vi "Configurable PWM Pulse Time Tester.vi"() -> ()   [LabVIEW 2021]
uses:
  <vilib>/Utility/error.llb/DialogType.ctl
  <vilib>/DAQmx/write.llb/DAQmx Write (Counter Frequency 1Chan 1Samp).vi
  <vilib>/DAQmx/create/channels.llb/DAQmx Create Channel (CO-Pulse Generation-Frequency).vi
  <vilib>/DAQmx/configure/timing.llb/DAQmx Timing (Implicit).vi
  <vilib>/DAQmx/miscellaneous.llb/DAQmx Fill In Error Info.vi
  <resource>/objmgr/daqmx.rc
panel:
  in  "stop":bool
  in  "Duty Cycle":dbl=5.0 min=5.0 max=10.0 format="%.6f"
  in  "Output Terminal":tag="/Dev1/PFI12"
  in  "Counter":tag="Dev1/ctr0"
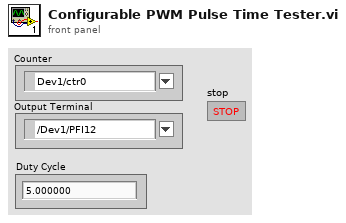
[diagram p1: front panel]
types:
  T1 = typedef "DialogType.ctl" = u16
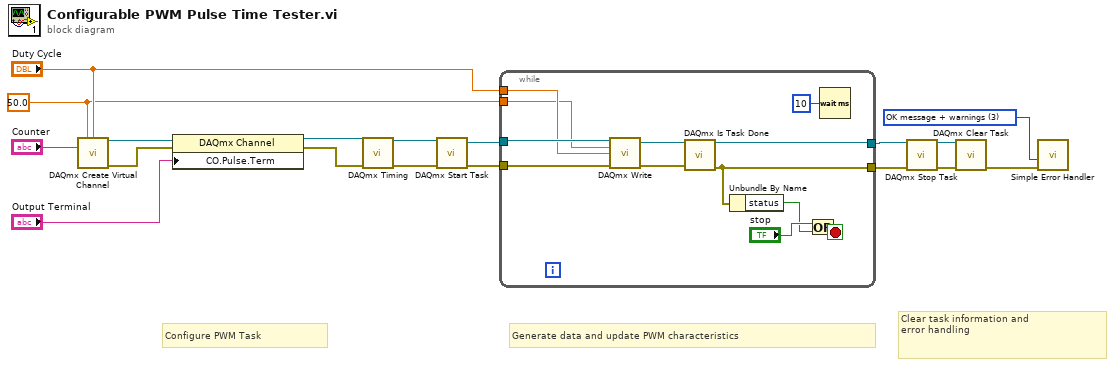
[diagram p0: block diagram]
diagram:
  w1 = 50.0 ("Frequency")
  w15 = T1 3 items=["no dialog", "OK message", "continue or stop message", "OK message + warnings", "continue/stop + warnings"] ("type of dialog (OK msg:1)")
  # "Clear task information and\nerror handling"
  # "Generate data and update PWM characteristics"
  # "Configure PWM Task"
  n1 = call-poly <vilib>:"DAQmx Create Virtual Channel.vi"("frequency"=w1, "duty cycle"="Duty Cycle", "counter"="Counter") -> ("task out"=w3:refnum<k21>, "error out"=w4:errorcluster)  [unwired: 11 in]
  n2 = property class="DAQmx Channel"(reference=w3, error in=w4, "CO.Pulse.Term"="Output Terminal") -> (reference out=w6:refnum<k21>, error out=w5:errorcluster)
  n3 = call-poly <vilib>:"DAQmx Timing.vi"("task/channels in"=w6, "error in"=w5) -> ("task out"=w9:refnum<k21>, "error out"=w8:errorcluster)  [unwired: 12 in]
  n4 = call <vilib>:"DAQmx Start Task.vi"("task/channels in"=w9, "error in"=w8) -> ("task out"=w13:refnum<k21>, "error out"=w12:errorcluster)  [unwired: 12 in]
  n5 = while {
    tunnel: w12 -> [w24]
    tunnel: [w27] -> w14
    tunnel: w13 -> [w23]
    tunnel: [w26] -> w11
    tunnel: "Duty Cycle" -> [w22]
    tunnel: w1 -> [w21]
    stop <- w29 stop-if-true
    n6 = call-poly <vilib>:"DAQmx Write.vi"("task/channels in"=w23, "frequency"=w21, "duty cycle"=w22, "error in"=w24) -> ("task out"=w19:refnum<k21>, "error out"=w20:errorcluster)  [unwired: 9 in, 1 out]
    n7 = call <vilib>:"DAQmx Is Task Done.vi"("task/channels in"=w19, "error in"=w20) -> ("task out"=w27:refnum<k21>, "error out"=w26:errorcluster)  [unwired: 11 in, 1 out]
    n8 = Unbundle By Name(w26) -> ("status"=w28:bool)
    n9 = Or(x="stop", y=w28) -> (x .or. y?=w29:bool)
    n10 = Wait (ms)(milliseconds to wait=u32 10) -> ()  [unwired: 1 out]
  }
  n11 = call <vilib>:"DAQmx Stop Task.vi"("task/channels in"=w14, "error in"=w11) -> ("task out"=w17:refnum<k21>, "error out"=w16:errorcluster)  [unwired: 12 in]
  n12 = call <vilib>:"DAQmx Clear Task.vi"("task in"=w17, "error in"=w16) -> ("error out"=w18:errorcluster)  [unwired: 13 in]
  n13 = call <vilib>:"Simple Error Handler.vi"("type of dialog (OK msg:1)"=w15, "error in (no error)"=w18) -> ()  [unwired: 3 in, 5 out]
